vi "TemplateQueueDriver.vi"(0 "State":string, 2 "Name":string, 5 "States[]":string[](array[string]), 7 "Data":variant, 11 "ErrorIn":errorcluster, 13 "Operation":T1) -> (4 "State":string, 8 "Data":variant, 15 "ErrorOut":errorcluster)   [LabVIEW 2018, in "ScreenGrabber.lvlib"]
uses:
  ScreenGrabber.lvlib
  Controls/QueueDriverStates.ctl
  Controls/QueueDriverDataType.ctl
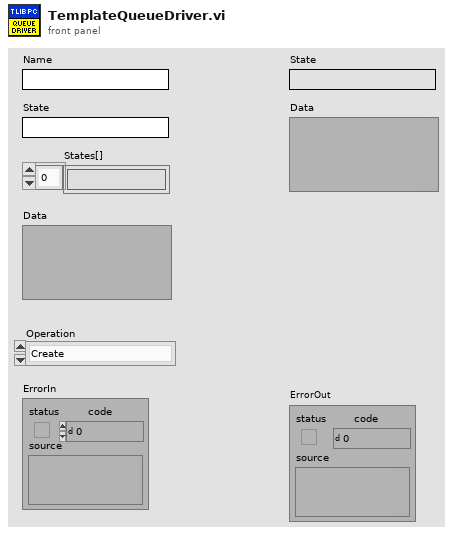
[diagram p1: front panel]
types:
  T1 = typedef "ScreenGrabber.lvlib/QueueDriverStates.ctl" = enum16{"Create", "Enqueue", "Enqueue N", "Dequeue", "Enstack", "Enstack N", "Flush", "Destroy"}
  T2 = typedef "ScreenGrabber.lvlib/QueueDriverDataType.ctl" = cluster{"State":string, "Data":variant}
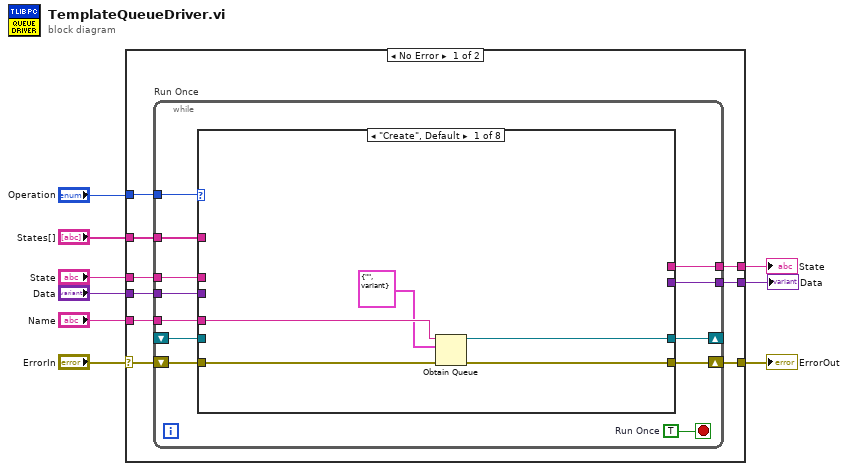
[diagram p0: block diagram]
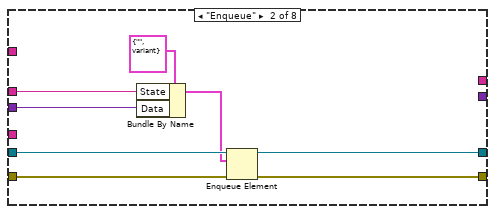
[diagram p2: hidden frame]
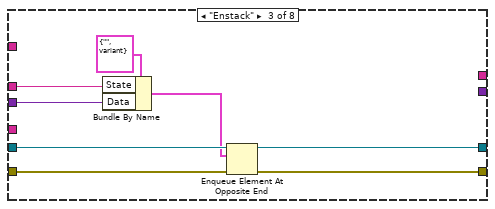
[diagram p3: hidden frame]
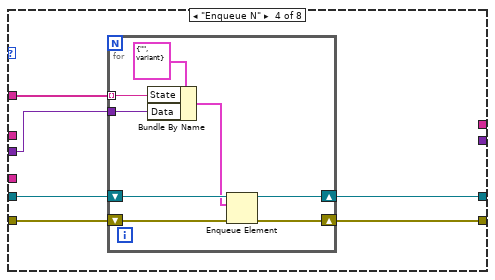
[diagram p4: hidden frame]
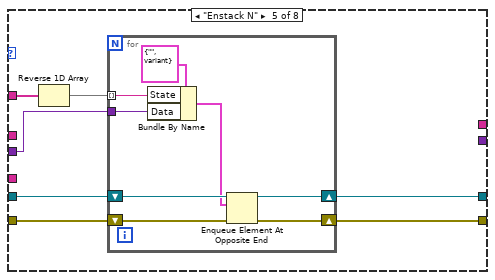
[diagram p5: hidden frame]
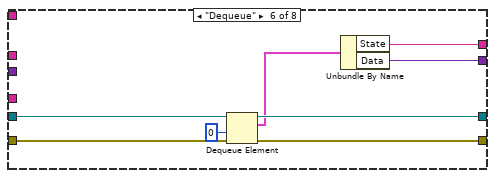
[diagram p6: hidden frame]
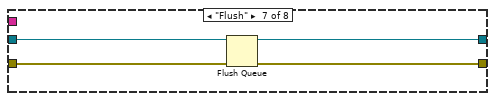
[diagram p7: hidden frame]
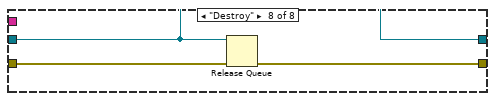
[diagram p8: hidden frame]
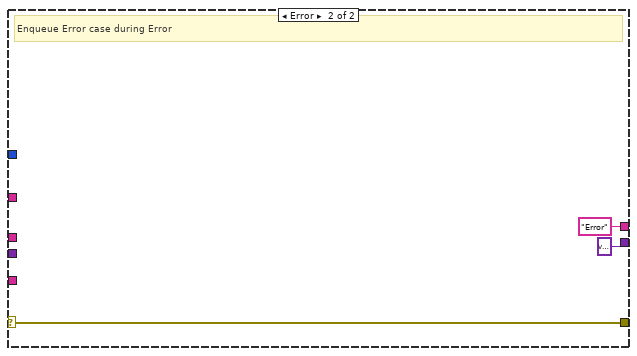
[diagram p9: hidden frame]
diagram:
  n1 = case shown="No Error" "ErrorIn" {
    selector: "ErrorIn" -> [w16 w98]
    tunnel: [w15 w98] -> w8
    tunnel: "Operation" -> [w18 _]
    tunnel: "Name" -> [w17 _]
    tunnel: "State" -> [w14 _]
    tunnel: "States[]" -> [w13 _]
    tunnel: [w12 "Error" ("Name")] -> w4
    tunnel: "Data" -> [w11 _]
    tunnel: [w10 variant ("Data")] -> w2
    frame No Error {
      n2 = while "Run Once" {
        tunnel: w18 -> [w30]
        tunnel: w17 -> [w29]
        shift-right: [w27] -> w15
        shift-left: w16 -> [w28]
        shift-right: [w25] -> _
        shift-left: _ -> [w24]
        tunnel: w14 -> [w23]
        tunnel: w13 -> [w22]
        tunnel: [w21] -> w12
        tunnel: w11 -> [w20]
        tunnel: [w19] -> w10
        stop <- w26 stop-if-true
        w26 = TRUE  # Run Once
        n3 = case shown="\"Create\", Default" w30 {
          tunnel: w29 -> [w35 _ _ _ _ _ _ _]
          tunnel: w28 -> [w34 w43 w51 w57 w72 w88 w89 w94]
          tunnel: [w33 w41 w49 w55 w70 w86 w91 w95] -> w27
          tunnel: [w32 w40 w48 w54 w69 w85 w90 w93] -> w25
          tunnel: w24 -> [_ w42 w50 w56 w71 w87 w92 w93]
          tunnel: w23 -> [_ w39 w47 _ _ _ _ _]
          tunnel: w22 -> [_ _ _ w53 w68 _ _ _]
          tunnel: [_ _ _ _ _ w82 _ _] -> w21
          tunnel: w20 -> [_ w37 w46 w52 w67 _ _ _]
          tunnel: [_ _ _ _ _ w81 _ _] -> w19
          frame "Create", Default {
            n4 = Obtain Queue(name (unnamed)=w35, element data type=T2 {"State"="", "Data"=variant} ("Cluster"), error in (no error)=w34) -> (queue out=w32:refnum<queue>, error out=w33:errorcluster)  [unwired: 2 in, 1 out]
          }
          frame "Enqueue" {
            n5 = Bundle By Name(cluster=T2 {"State"="", "Data"=variant} ("Cluster"), "State"=w39, "Data"=w37) -> (w38:T2)
            n6 = Enqueue Element(queue=w42, element=w38, error in (no error)=w43) -> (queue out=w40:refnum<queue>, error out=w41:errorcluster)  [unwired: 1 in, 1 out]
          }
          frame "Enstack" {
            n7 = Bundle By Name(cluster=T2 {"State"="", "Data"=variant} ("Cluster"), "State"=w47, "Data"=w46) -> (w45:T2)
            n8 = Enqueue Element At Opposite End(queue=w50, element=w45, error in (no error)=w51) -> (queue out=w48:refnum<queue>, error out=w49:errorcluster)  [unwired: 1 in, 1 out]
          }
          frame "Enqueue N" {
            n9 = for {
              tunnel: w53 -> [w61] mode=indexing
              shift-right: [w63] -> w55
              shift-left: w57 -> [w65]
              shift-right: [w62] -> w54
              shift-left: w56 -> [w64]
              tunnel: w52 -> [w60]
              n10 = Bundle By Name(cluster=T2 {"State"="", "Data"=variant} ("Cluster"), "State"=w61, "Data"=w60) -> (w59:T2)
              n11 = Enqueue Element(queue=w64, element=w59, error in (no error)=w65) -> (queue out=w62:refnum<queue>, error out=w63:errorcluster)  [unwired: 1 in, 1 out]
            }
          }
          frame "Enstack N" {
            n12 = Reverse 1D Array(array=w68) -> (reversed array=w66:string[])
            n13 = for {
              tunnel: w66 -> [w76] mode=indexing
              shift-right: [w78] -> w70
              shift-left: w72 -> [w80]
              shift-right: [w77] -> w69
              shift-left: w71 -> [w79]
              tunnel: w67 -> [w75]
              n14 = Bundle By Name(cluster=T2 {"State"="", "Data"=variant} ("Cluster"), "State"=w76, "Data"=w75) -> (w74:T2)
              n15 = Enqueue Element At Opposite End(queue=w79, element=w74, error in (no error)=w80) -> (queue out=w77:refnum<queue>, error out=w78:errorcluster)  [unwired: 1 in, 1 out]
            }
          }
          frame "Dequeue" {
            n16 = Dequeue Element(queue=w87, timeout in ms (-1)=0, error in (no error)=w88) -> (queue out=w85:refnum<queue>, element=w83:T2, error out=w86:errorcluster)  [unwired: 1 out]
            n17 = Unbundle By Name(w83) -> ("State"=w82:string, "Data"=w81:variant)
          }
          frame "Flush" {
            n18 = Flush Queue(queue=w92, error in (no error)=w89) -> (queue out=w90:refnum<queue>, error out=w91:errorcluster)  [unwired: 1 out]
          }
          frame "Destroy" {
            n19 = Release Queue(queue=w93, error in (no error)=w94) -> (error out=w95:errorcluster)  [unwired: 1 in, 2 out]
          }
        }
      }
    }
    frame Error {
      # "Enqueue Error case during Error"
    }
  }
  "ErrorOut" <- w8
  "State" <- w4
  "Data" <- w2
